vi "GetPrice.vi"(8 "error in (no error)":errorcluster, 11 "TV in":refnum<class "TV.lvclass">) -> (0 "error out":errorcluster, 2 "Price":dbl, 3 "TV out":refnum<class "TV.lvclass">)   [LabVIEW 2019, in "TV.lvclass"]
uses:
  TV.lvclass
  Furniture.lvclass
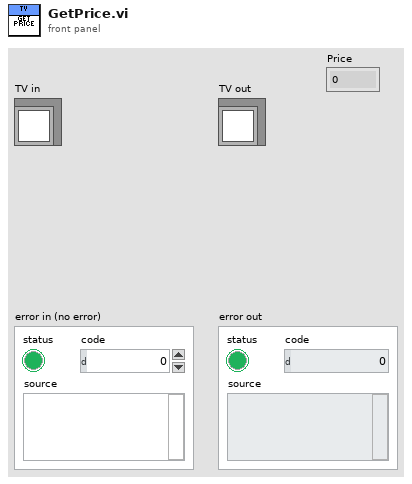
[diagram p1: front panel]
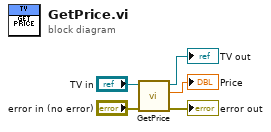
[diagram p0: block diagram]
diagram:
  n1 = call-parent "GetPrice.vi"("error in (no error)"="error in (no error)", "Furniture in"="TV in") -> ("error out"=→"error out":errorcluster, "Price"=→"Price":dbl, "Furniture out"=→"TV out":refnum<class "TV.lvclass">)  [unwired: 7 in]
